vi "Set Up Dialog - Light & Laser.vi"() -> ()   [LabVIEW 2012]
panel:
  out "Calibration Instructions":string="1. Connect the sensor to your myDAQ as shown in the diagram above.\n\n2. Connect two sets of LSN-100's Light & Laser sensors to both channels of the IX-MYDAQ.\n\n3. Connect the NI myDAQ to your computer using a USB cable."
  # "iWorx - Light & Laser - Set Up"
  # "Light Sensor & Laser x 2 (LSN-100)"
  # "iWorx"
  # "Sensor"
  # "LSN - 100"
  # "myDAQ"
  # "Computer"
  # "Adaptor"
  # "Connection Diagram"
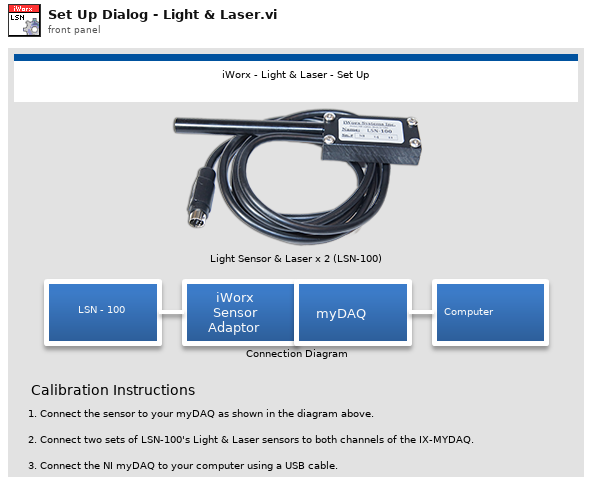
[diagram p1: front panel]
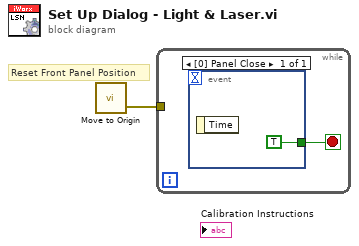
[diagram p0: block diagram]
diagram:
  # "Reset Front Panel Position"
  n1 = call "Move to Origin.vi"() -> ("Error Out"=w1:errorcluster)  [unwired: 3 in]
  n2 = while {
    tunnel: w1 -> [_]
    stop <- w2 stop-if-true
    n3 = event shown="[0] Panel Close" {
      selector: _ -> [_]
      dyn-events: _ -> [_]
      timeout: _ -> [_]
      tunnel: [TRUE] -> w2
      event Panel Close {
        n4 = event-data() -> ()  [unwired: 1 in, 1 out]
      }
    }
  }
